vi "Teleop.vi"(10 "Match Info":T1={"Autonomous Elapsed Seconds"=0.0, "TeleOp Elapsed Seconds"=84.436, "Disabled Elapsed Seconds"=0.0, "Visited Autonomous"=FALSE, "Visited TeleOp"=TRUE, "Visited Disabled"=FALSE, "Autonomous Settings"={"Autonomous Style"=enum."Independent", "VI Refnum"=refnum}}, 11 "Call Context":T2=enum."Execute") -> ()   [LabVIEW 2011]
doc: "This VI is called for each TeleOp packet received from the DS where the robot is not disabled. It is often used to read from the joysticks and update I/O or to update setpoints for timed control loops. It should complete and return within 20 milliseconds or it may miss DS packets."
uses:
  <vilib>/Rock Robotics/WPI/DriverStation/WPI_DriverStationDerivedRobotMode.ctl
  <vilib>/Rock Robotics/WPI/DriverStation/WPI_DriverStationMatch Info.ctl
  Controls/Jaguar Control Modes.ctl
  Robot Global Data.vi
  Globals/Jaguar Control Mode.vi
  Globals/Are We Calibrating Steering.vi
  Autonomous/Auto Drive Emulation.vi
  Globals/Autonomous Tipping.vi
  Globals/Jaguar Commands.vi
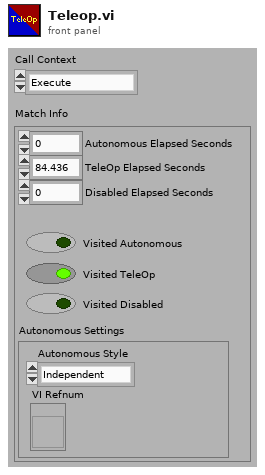
[diagram p1: front panel]
types:
  T1 = typedef "WPI_DriverStationMatch Info.ctl" = cluster{"Autonomous Elapsed Seconds":dbl, "TeleOp Elapsed Seconds":dbl, "Disabled Elapsed Seconds":dbl, "Visited Autonomous":bool, "Visited TeleOp":bool, "Visited Disabled":bool, "Autonomous Settings":cluster{"Autonomous Style":enum16{"Iterative", "Independent"}, "VI Refnum":refnum<vi>}}
  T2 = typedef "WPI_DriverStationDerivedRobotMode.ctl" = enum16{"Init", "Execute", "Stop"}
  T3 = typedef "Jaguar Control Modes.ctl" = enum16{"Speed", "Position"}
  T4 = typedef "Robot Orientation.ctl" = enum16{"Landscape", "Portrait"}
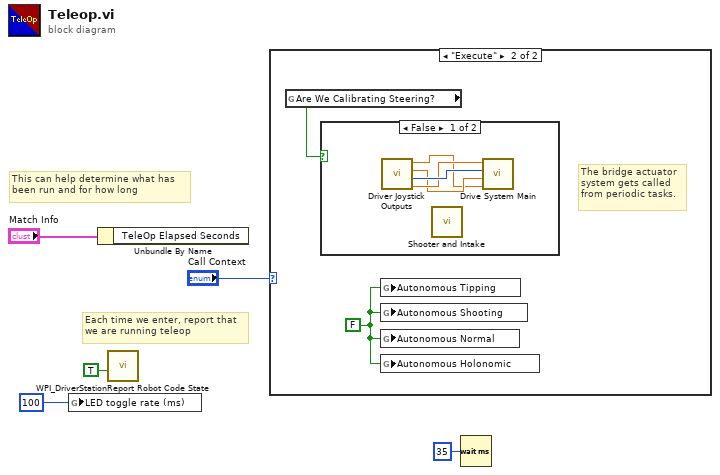
[diagram p0: block diagram]
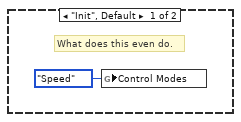
[diagram p2: hidden frame]
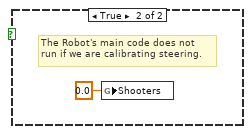
[diagram p3: hidden frame]
diagram:
  # "Each time we enter, report that\nwe are running teleop"
  # "This can help determine what has\nbeen run and for how long"
  n1 = global write "Robot Global Data.vi" "LED toggle rate (ms)"(u32 100 ("LED ms toggle rate")) -> ()
  n2 = Unbundle By Name("Match Info") -> ()  [unwired: 1 out]
  n3 = call <vilib>:"WPI_DriverStationReport Robot Code State.vi"("TeleOp"=TRUE ("Autonomous")) -> ()  [unwired: 10 in, 1 out]
  n4 = case shown="\"Execute\"" "Call Context" {
    frame "Init", Default {
      # "What does this even do."
      n5 = global write "Jaguar Control Mode.vi" "Control Modes"(Jaguar_Control_Modes."Speed" ("Mode")) -> ()
    }
    frame "Execute" {
      w7 = FALSE ("Autonomous Tipping")
      # "The bridge actuator\nsystem gets called\nfrom periodic tasks."
      n6 = global read "Are We Calibrating Steering.vi" "Are We Calibrating Steering?"() -> (w8:bool)
      n7 = case shown="False" w8 {
        frame False {
          n8 = call "Driver Joystick Outputs.vi"() -> ("Joy X"=w9:dbl, "Joy Y"=w10:dbl, "Robot Orientation"=w12:T4, "Joy Twist"=w11:dbl)  [unwired: 3 in]
          n9 = call "Shooter and Intake.vi"() -> ()  [unwired: 1 in]
          n10 = call "Drive System Main.vi"("Joy X"=w9, "Joy Y"=w10, "Robot Orientation"=w12, "Joy Twist"=w11) -> ()  [unwired: 8 in]
        }
        frame True {
          # "The Robot's main code does not \nrun if we are calibrating steering."
          n11 = global write "Jaguar Commands.vi" "Shooters"(0.0 ("Shooters")) -> ()
        }
      }
      n12 = global write "Autonomous Tipping.vi" "Autonomous Tipping"(w7) -> ()
      n13 = global write "Auto Drive Emulation.vi" "Autonomous Shooting"(w7) -> ()
      n14 = global write "Auto Drive Emulation.vi" "Autonomous Normal"(w7) -> ()
      n15 = global write "Auto Drive Emulation.vi" "Autonomous Holonomic"(w7) -> ()
    }
  }
  n16 = Wait (ms)(milliseconds to wait=u32 35) -> ()  [unwired: 1 out]
